vi "Matrix Copy Print Result.vi"() -> ()   [LabVIEW 2014, in "Arduino MatrixMath.lvlib"]
uses:
  <vilib>/Aledyne-TSXperts/Arduino Compatible Compiler for LabVIEW/addons/Arduino MatrixMath/Arduino MatrixMath.lvlib
  <vilib>/Aledyne-TSXperts/Arduino Compatible Compiler for LabVIEW/Arduino Compatible Compiler for LabVIEW.lvlib
panel:
  in  "A":sgl[](array[numeric])=[1.0, 2.0, 3.0, 4.0, 5.0, 6.0, 7.0, 8.0]
  out "Error Out":errorcluster
  in  "Error In":errorcluster
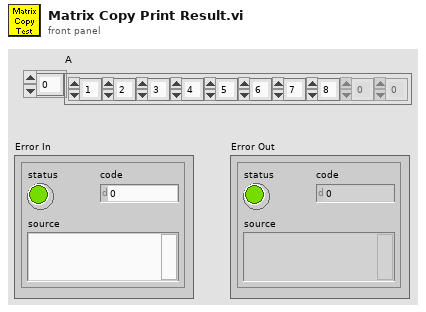
[diagram p1: front panel]
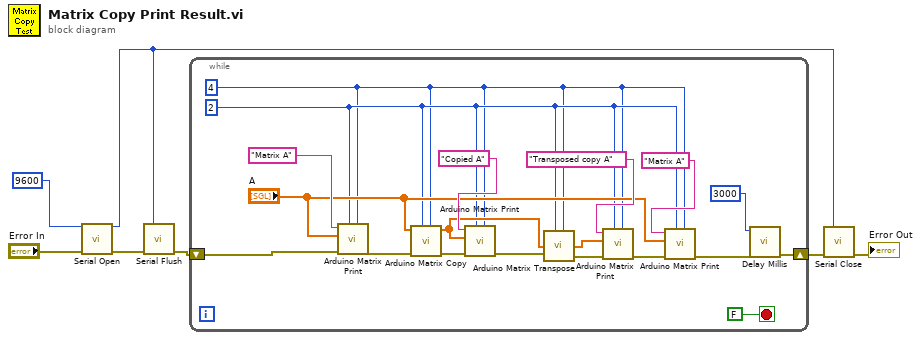
[diagram p0: block diagram]
diagram:
  n1 = call <vilib>:"Serial Open.vi"("Speed"=u32 9600, "error in (no error)"="Error In") -> ("Instance"=w1:u8, "error out"=w3:errorcluster)  [unwired: 12 in]
  n2 = call <vilib>:"Serial Flush.vi"("Instance"=w1, "error in (no error)"=w3) -> ("error out"=w2:errorcluster)  [unwired: 13 in]
  n3 = while {
    shift-right: [w23] -> w7
    shift-left: w2 -> [w25]
    stop <- FALSE stop-if-true
    w8 = u8 4 ("cols num.")
    w9 = u8 2 ("rows num.")
    n4 = call <vilib>:"Arduino Matrix Print.vi"("cols num."=w8, "rows num."=w9, "Error In"=w25, "A"="A", "Label"="Matrix A") -> ("Error Out"=w21:errorcluster)  [unwired: 6 in]
    n5 = call <vilib>:"Arduino Matrix Copy.vi"("cols num."=w8, "rows num."=w9, "Error In"=w21, "A"="A") -> ("Error Out"=w20:errorcluster, "A copy"=w18:sgl[])  [unwired: 6 in]
    n6 = call <vilib>:"Arduino Matrix Print.vi"("cols num."=w8, "rows num."=w9, "Error In"=w20, "A"=w18, "Label"="Copied A") -> ("Error Out"=w17:errorcluster)  [unwired: 6 in]
    n7 = call <vilib>:"Arduino Matrix Transpose.vi"("rows num."=w9, "A"=w18, "Error In"=w17, "cols num."=w8) -> ("transposed A"=w15:sgl[], "Error Out"=w16:errorcluster)  [unwired: 4 in]
    n8 = call <vilib>:"Arduino Matrix Print.vi"("cols num."=w8, "rows num."=w9, "Error In"=w16, "A"=w15, "Label"="Transposed copy A") -> ("Error Out"=w13:errorcluster)  [unwired: 6 in]
    n9 = call <vilib>:"Arduino Matrix Print.vi"("cols num."=w8, "rows num."=w9, "Error In"=w13, "A"="A", "Label"="Matrix A") -> ("Error Out"=w12:errorcluster)  [unwired: 6 in]
    n10 = call <vilib>:"Delay Millis.vi"("error in (no error)"=w12, "delay"=u32 3000) -> ("error out"=w23:errorcluster)  [unwired: 9 in]
  }
  n11 = call <vilib>:"Serial Close.vi"("Instance"=w1, "error in (no error)"=w7) -> ("error out"=→"Error Out":errorcluster)  [unwired: 13 in]
